vi "Simple Mediator Pattern.vi"() -> ()   [LabVIEW 2016, in "Stream Mediator.lvlib"]
doc: "--\nCopyright © 2017 Composed SystemsI All rights reserved.\n\nAuthor: Jon McBee <jon.mcbee@composed.io>\n\nThis library is provided \"AS IS\" ,WITHOUT WARRANTIES OR\nCONDITIONS OF ANY KIND, either express or implied.\n\nComposed Systems -- composed.io\n\nStream 0.0.1.1\nJon McBee - Composed Systems\nCopyright (c) 2017, Composed Systems"
uses:
  <userlib>/Composed Systems/Stream/Mediator/Stream Mediator.lvlib
  <vilib>/Composed Systems/Stream/Mediator/Classes/Message Broker Interface Ref/Message Broker Interface Ref.lvclass
  <vilib>/Composed Systems/Stream/Mediator/Classes/Message Double/Message Double.lvclass
  <vilib>/Composed Systems/Stream/Mediator/Classes/Message Transport Queue/Message Transport Queue.lvclass
  <vilib>/Composed Systems/Stream/Mediator/Classes/Message Transport Event/Message Transport Event.lvclass
  <vilib>/Composed Systems/Stream/Mediator/Example/Example Actor/Example Actor.lvclass
  <vilib>/ActorFramework/Actor/Actor.lvclass
  <vilib>/Composed Systems/Stream/Mediator/Classes/Message Transport Singleton/Message Transport Singleton.lvclass
  <vilib>/ActorFramework/Stop Msg/Stop Msg.lvclass
panel:
  in  "Get Singleton":bool
  out "Data S":dbl
  out "Data B":dbl
  out "Data E":dbl
  out "Data Q":dbl
  in  "Data":dbl
  in  "Publish Rate":u32=100
  in  "stop":bool
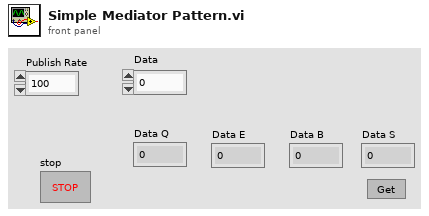
[diagram p1: front panel]
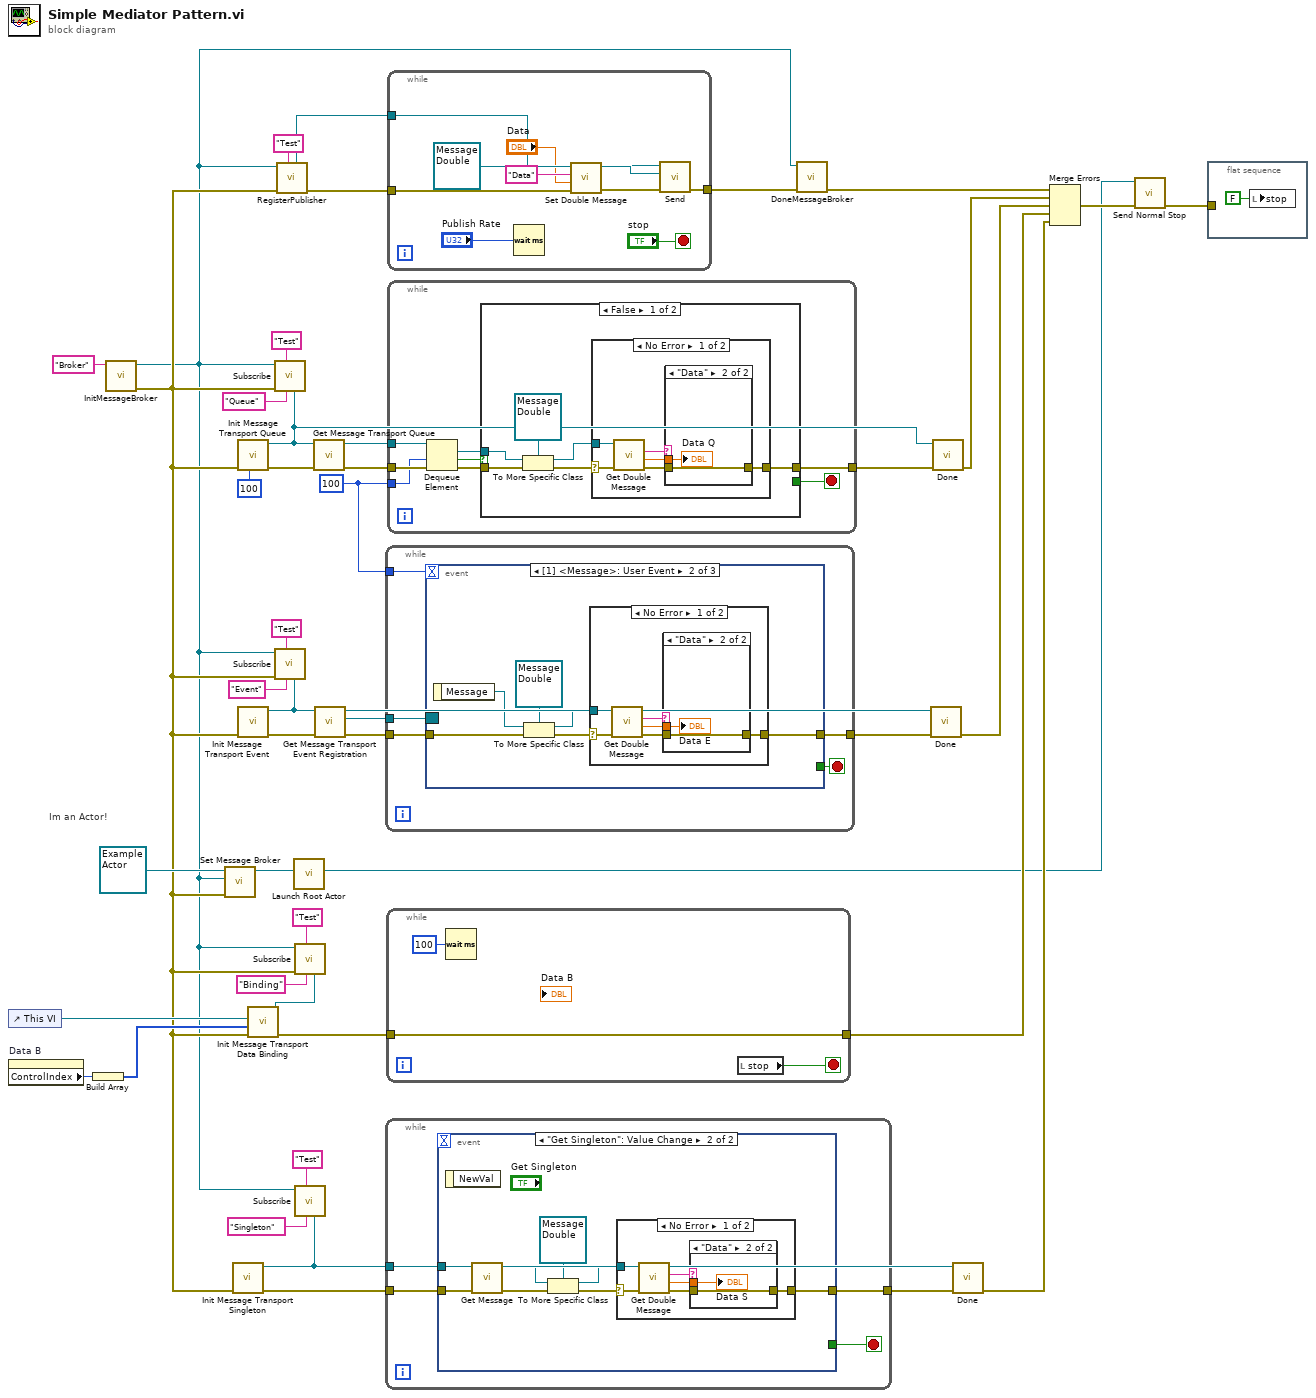
[diagram p0: block diagram]
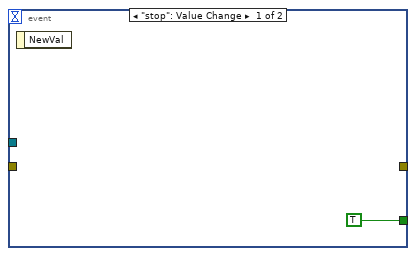
[diagram p2: hidden frame]
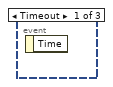
[diagram p5: hidden frame]
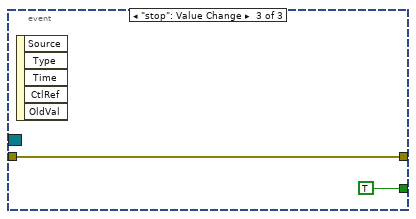
[diagram p8: hidden frame]
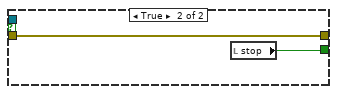
[diagram p11: hidden frame]
diagram:
  w34 = 100 ("timeout in ms (-1)")
  # "Im an Actor!"
  n1 = control-ref of="This VI"() -> (w18:refnum<vi>)
  n2 = property on="Data B" class="DigNum (strict)"() -> ("ControlIndex"=w15:i32)  [unwired: 2 in, 2 out]
  n3 = Build Array(w15) -> (w14:i32[])
  n4 = call <vilib>:"InitMessageBroker.vi"("Broker Name"="Broker") -> ("error out"=w9:errorcluster, "Message Broker Interface Ref out"=w1:refnum<class "Message Broker Interface Ref.lvclass">)  [unwired: 9 in]
  n5 = call <vilib>:"Set Message Broker.vi"("error in (no error)"=w9, "Message Broker"=w1, "Example Actor in"=refnum<class "Example Actor.lvclass"> refnum ("Example Actor.lvclass")) -> ("Example Actor out"=w12:refnum<class "Example Actor.lvclass">)  [unwired: 7 in, 1 out]
  n6 = call <vilib>:"Init Message Transport Singleton.vi"("error in (no error)"=w9) -> ("error out"=w8:errorcluster, "Message Transport Singleton out"=w5:refnum<class "Message Transport Singleton.lvclass">)  [unwired: 9 in]
  n7 = call <vilib>:"Init Message Transport Queue.vi"("Max Queue Size"=100, "error in (no error)"=w9) -> ("error out"=w39:errorcluster, "Message Transport Queue out"=w30:refnum<class "Message Transport Queue.lvclass">)  [unwired: 8 in]
  n8 = call <vilib>:"Init Message Transport Event.vi"("error in (no error)"=w9) -> ("error out"=w36:errorcluster, "Message Transport Event out"=w42:refnum<class "Message Transport Event.lvclass">)  [unwired: 9 in]
  n9 = call <vilib>:"Init Message Transport Data Binding.vi"("error in (no error)"=w9, "Control Indexes"=w14, "VI Refnum"=w18) -> ("error out"=w17:errorcluster, "Message Transport Binding out"=w21:refnum<class "Message Transport Binding.lvclass">)  [unwired: 7 in]
  n10 = call-dynamic "Subscribe.vi"("Message Transport Interface"=w30, "Subscriber Name"="Queue", "Topic Name"="Test", "error in (no error)"=w9, "Message Broker Interface TAP in"=w1) -> ()  [unwired: 4 in, 3 out]
  n11 = call-dynamic "Subscribe.vi"("Message Transport Interface"=w42, "Subscriber Name"="Event", "Topic Name"="Test", "error in (no error)"=w9, "Message Broker Interface TAP in"=w1) -> ()  [unwired: 4 in, 3 out]
  n12 = call-dynamic "RegisterPublisher.vi"("Topic Name"="Test", "error in (no error)"=w9, "Message Broker Interface Ref in"=w1) -> ("error out"=w41:errorcluster, "Transport"=w40:refnum<class "Message Transport Queue.lvclass">)  [unwired: 4 in, 3 out]
  n13 = call <vilib>:"Launch Root Actor.vi"("Actor"=w12) -> ("Actor's Enqueuer"=w2:refnum<class "Message Enqueuer.lvclass">)  [unwired: 9 in, 1 out]
  n14 = call-dynamic "Subscribe.vi"("Message Transport Interface"=w21, "Subscriber Name"="Binding", "Topic Name"="Test", "error in (no error)"=w9, "Message Broker Interface TAP in"=w1) -> ()  [unwired: 4 in, 3 out]
  n15 = call-dynamic "Subscribe.vi"("Message Transport Interface"=w5, "Subscriber Name"="Singleton", "Topic Name"="Test", "Message Broker Interface TAP in"=w1) -> ()  [unwired: 5 in, 3 out]
  n16 = call <vilib>:"Get Message Transport Queue.vi"("error in (no error)"=w39, "Message Transport Queue in"=w30) -> ("error out"=w38:errorcluster, "Queue"=w37:refnum<queue>)  [unwired: 8 in]
  n17 = call <vilib>:"Get Message Transport Event Registration.vi"("error in (no error)"=w36, "Message Transport Event in"=w42) -> ("error out"=w35:errorcluster, "Event Registration Refnum"=w23:refnum<event-registration>, "Message Transport Event out"=w31:refnum<class "Message Transport Event.lvclass">)  [unwired: 6 in, 1 out]
  n18 = while {
    tunnel: w23 -> [w51]
    tunnel: w35 -> [w50]
    tunnel: [w49] -> w32
    tunnel: w34 -> [w48]
    stop <- w47 stop-if-true
    n19 = event shown="[1] <Message>: User Event" {
      selector: w51 -> [_ _ _]
      dyn-events: _ -> [_ _ _]
      timeout: w48 -> [_ _ _]
      tunnel: w50 -> [_ w56 w69]
      tunnel: [_ w52 w69] -> w49
      tunnel: [_ _ TRUE] -> w47
      event Timeout {
        n20 = event-data() -> ()  [unwired: 1 in, 1 out]
      }
      event User Event {
        n21 = event-data() -> ("Message"=w55:refnum<class "Message Interface.lvclass">)  [unwired: 1 in]
        n22 = To More Specific Class(target class=refnum<class "Message Double.lvclass"> refnum ("Message Double.lvclass"), reference=w55, error in=w56) -> (specific class reference=w53:refnum<class "Message Double.lvclass">, error out=w54:errorcluster)
        n23 = case shown="No Error" w54 {
          selector: w54 -> [w63 w67]
          tunnel: [w58 w67] -> w52
          tunnel: w53 -> [w62 _]
          frame No Error {
            n24 = call <vilib>:"Get Double Message.vi"("error in (no error)"=w63, "Message Double in"=w62) -> ("error out"=w59:errorcluster, "Value"=w60:dbl, "Name"=w61:string)  [unwired: 6 in, 1 out]
            n25 = case shown="\"Data\"" w61 {
              tunnel: w60 -> [_ w65]
              tunnel: w59 -> [w64 w66]
              tunnel: [w64 w66] -> w58
              frame Default {
              }
              frame "Data" {
                "Data E" <- w65
              }
            }
          }
          frame Error {
          }
        }
      }
      event "stop": Value Change {
        n26 = event-data() -> ()  [unwired: 1 in, 5 out]
      }
    }
  }
  n27 = while {
    tunnel: w8 -> [w71]
    tunnel: [w70] -> w6
    tunnel: w5 -> [w72]
    stop <- w73 stop-if-true
    n28 = event shown="[1] \"Get Singleton\": Value Change" {
      selector: _ -> [_ _]
      dyn-events: _ -> [_ _]
      timeout: _ -> [_ _]
      tunnel: [TRUE _] -> w73
      tunnel: w72 -> [_ w82]
      tunnel: w71 -> [_ w76]
      tunnel: [_ w75] -> w70
      event "stop": Value Change {
        n29 = event-data() -> ()  [unwired: 1 in, 1 out]
      }
      event "Get Singleton": Value Change {
        n30 = event-data() -> ()  [unwired: 1 in, 1 out]
        n31 = call <vilib>:"Get Message.vi"("error in (no error)"=w76, "Message Transport Singleton in"=w82) -> ("error out"=w78:errorcluster, "Message"=w77:refnum<class "Message Interface.lvclass">)  [unwired: 8 in]
        n32 = To More Specific Class(target class=refnum<class "Message Double.lvclass"> refnum ("Message Double.lvclass"), reference=w77, error in=w78) -> (specific class reference=w79:refnum<class "Message Double.lvclass">, error out=w80:errorcluster)
        n33 = case shown="No Error" w80 {
          selector: w80 -> [w88 w92]
          tunnel: [w83 w92] -> w75
          tunnel: w79 -> [w87 _]
          frame No Error {
            n34 = call <vilib>:"Get Double Message.vi"("error in (no error)"=w88, "Message Double in"=w87) -> ("error out"=w84:errorcluster, "Value"=w85:dbl, "Name"=w86:string)  [unwired: 6 in, 1 out]
            n35 = case shown="\"Data\"" w86 {
              tunnel: w85 -> [_ w90]
              tunnel: w84 -> [w89 w91]
              tunnel: [w89 w91] -> w83
              frame Default {
              }
              frame "Data" {
                "Data S" <- w90
              }
            }
          }
          frame Error {
          }
        }
      }
    }
  }
  n36 = while {
    tunnel: w17 -> [w93]
    tunnel: [w93] -> w16
    stop <- w95 stop-if-true
    n37 = Wait (ms)(milliseconds to wait=u32 100) -> ()  [unwired: 1 out]
    n38 = local read "stop"() -> (w95:bool)
  }
  n39 = while {
    tunnel: w41 -> [w103]
    tunnel: w40 -> [w97]
    tunnel: [w96] -> w29
    stop <- "stop" stop-if-true
    n40 = Wait (ms)(milliseconds to wait="Publish Rate") -> ()  [unwired: 1 out]
    n41 = call <vilib>:"Set Double Message.vi"("error in (no error)"=w103, "Value"="Data", "Name"="Data", "Message Double in"=refnum<class "Message Double.lvclass"> refnum ("Message Double.lvclass")) -> ("error out"=w99:errorcluster, "Message Double out"=w98:refnum<class "Message Double.lvclass">)  [unwired: 6 in]
    n42 = call-dynamic "Send.vi"("error in (no error)"=w99, "Message"=w98, "Message Transport Queue in"=w97) -> ("error out"=w96:errorcluster)  [unwired: 6 in, 2 out]
  }
  n43 = while {
    tunnel: w38 -> [w112]
    tunnel: w37 -> [w113]
    tunnel: w34 -> [w111]
    tunnel: [w106] -> w33
    stop <- w107 stop-if-true
    n44 = Dequeue Element(queue=w113, timeout in ms (-1)=w111, error in (no error)=w112) -> (element=w109:refnum<class "Message Interface.lvclass">, timed out?=w110:bool, error out=w108:errorcluster)  [unwired: 1 out]
    n45 = case shown="False" w110 {
      tunnel: w109 -> [w119 _]
      tunnel: w108 -> [w118 w131]
      tunnel: [w115 w131] -> w106
      tunnel: [_ w130] -> w107
      frame False {
        n46 = To More Specific Class(target class=refnum<class "Message Double.lvclass"> refnum ("Message Double.lvclass"), reference=w119, error in=w118) -> (specific class reference=w114:refnum<class "Message Double.lvclass">, error out=w116:errorcluster)
        n47 = case shown="No Error" w116 {
          selector: w116 -> [w125 w129]
          tunnel: [w120 w129] -> w115
          tunnel: w114 -> [w124 _]
          frame No Error {
            n48 = call <vilib>:"Get Double Message.vi"("error in (no error)"=w125, "Message Double in"=w124) -> ("error out"=w121:errorcluster, "Value"=w122:dbl, "Name"=w123:string)  [unwired: 6 in, 1 out]
            n49 = case shown="\"Data\"" w123 {
              tunnel: w122 -> [_ w127]
              tunnel: w121 -> [w126 w128]
              tunnel: [w126 w128] -> w120
              frame Default {
              }
              frame "Data" {
                "Data Q" <- w127
              }
            }
          }
          frame Error {
          }
        }
      }
      frame True {
        n50 = local read "stop"() -> (w130:bool)
      }
    }
  }
  n51 = call <vilib>:"DoneMessageBroker.vi"("error in (no error)"=w29, "Message Broker Interface Ref in"=w1) -> ("error out"=w28:errorcluster)  [unwired: 8 in, 1 out]
  n52 = call-dynamic "Done.vi"("error in (no error)"=w32, "Message Transport Event in"=w31) -> ("error out"=w26:errorcluster)  [unwired: 8 in, 1 out]
  n53 = call-dynamic "Done.vi"("error in (no error)"=w33, "Message Transport Queue in"=w30) -> ("error out"=w27:errorcluster)  [unwired: 8 in, 1 out]
  n54 = call-dynamic "Done.vi"("error in (no error)"=w6, "Message Transport Singleton in"=w5) -> ("error out"=w7:errorcluster)  [unwired: 8 in, 1 out]
  n55 = Merge Errors(w28, w27, w26, w16, w7) -> (w4:errorcluster)
  n56 = call <vilib>:"Send Normal Stop.vi"("error in (no error)"=w4, "Message Enqueuer"=w2) -> ("error out"=w3:errorcluster)  [unwired: 9 in]
  n57 = flat-sequence {
    tunnel: w3 -> [_]
    frame #0 {
      n58 = local write "stop"(FALSE ("stop")) -> ()
    }
  }
